vi "Get Type Name.vi"(11 "Instrument in":refnum<class "Instrument.lvclass">) -> (2 "Type Name":string)   [LabVIEW 2019, in "Instrument.lvlib" / "Instrument.lvclass"]
uses:
  Instrument.lvclass
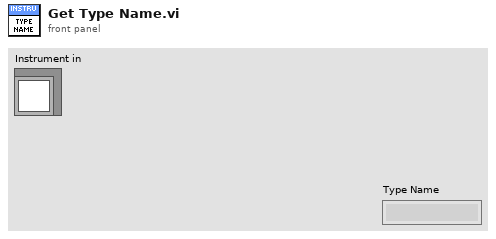
[diagram p1: front panel]
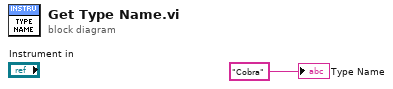
[diagram p0: block diagram]
diagram:
  "Type Name" <- "Cobra" ("Type Name")
